vi "USBWhrite.vi"(8 "error in (no error)":errorcluster, 10 "Bulk Out Data:":string="*IDN?\n", 11 "USB":refnum<visa-resource-name>="USB0::0x1043::0x0000::NI-VISA-0::RAW") -> (0 "error out":errorcluster, 3 "VISA Resource Name":refnum<visa-resource-name>)   [LabVIEW 2011]
doc: "The vi are writing information to the specified USB connection."
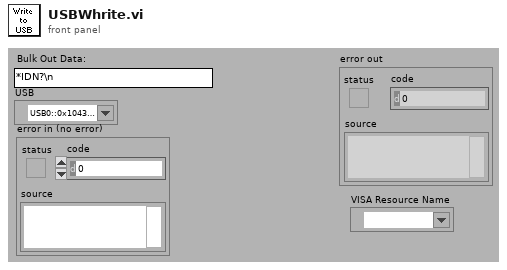
[diagram p1: front panel]
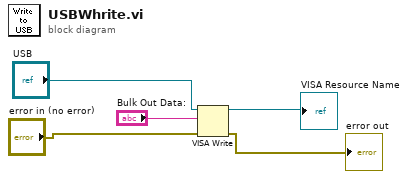
[diagram p0: block diagram]
diagram:
  n1 = VISA Write(VISA resource name="USB", write buffer="Bulk Out Data:", error in (no error)="error in (no error)") -> (VISA resource name out=→"VISA Resource Name":refnum<visa-resource-name>, error out=→"error out":errorcluster)  [unwired: 1 out]
